vi "UpdateFileName (SubVI).vi"(9 "File Extension":string, 10 "Append to Filename":string, 11 "Path and filename":path) -> (3 "Updated Path":path)   [LabVIEW 2016]
uses:
  <vilib>/regexp/Match Regular Expression.xnode
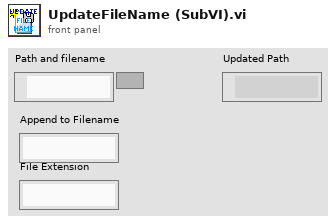
[diagram p1: front panel]
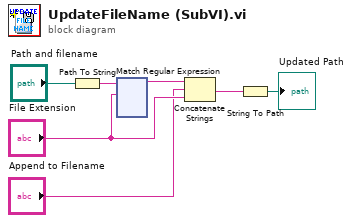
[diagram p0: block diagram]
diagram:
  n1 = Path To String(path="Path and filename") -> (string=w2:string)
  n2 = xnode "Match Regular Expression"("input string"=w2, "regular expression"="File Extension") -> ("before match"=w4:string)  [unwired: 4 in, 4 out]
  n3 = Concatenate Strings(w4, "Append to Filename", "File Extension") -> (w5:string)
  n4 = String To Path(string=w5) -> (path=→"Updated Path":path)
